vi "CreateVIA.vi"() -> (3 "VIA out":refnum<class "VIA.lvclass">)   [LabVIEW 2012, in "VIAManager.lvclass"]
uses:
  <vilib>/NXT/LegoClasses/BrickManagers/VIAManager/VIAManager.lvclass
  <vilib>/NXT/LegoClasses/VIA/VIA.lvclass
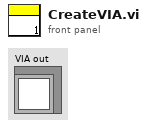
[diagram p1: front panel]
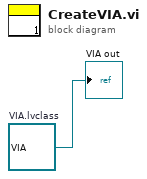
[diagram p0: block diagram]
diagram:
  w1 = refnum<class "VIA.lvclass"> refnum  # VIA.lvclass
  "VIA out" <- w1
